vi "Read Properties.vi"(11 "Grid in":refnum<class "Grid.lvclass">) -> (0 "No Neurons":i32, 1 "Neurons Info":T1, 2 "Size(um)":u32[](array[numeric]), 3 "Grid out":refnum<class "Grid.lvclass">, 4 "Created at":timestamp, 5 "Name XML File":string, 6 "Comments":string, 7 "Path":path)   [LabVIEW 2013, in "Grid.lvclass"]
doc: "This VI gets the global information of the grid: No Neurons, Neurons Info, and Size Cube"
uses:
  Grid.lvclass
  Controls/Neuron Info.ctl
  Controls/Type of Neuron.ctl
  Grid.lvclass/Grid.ctl
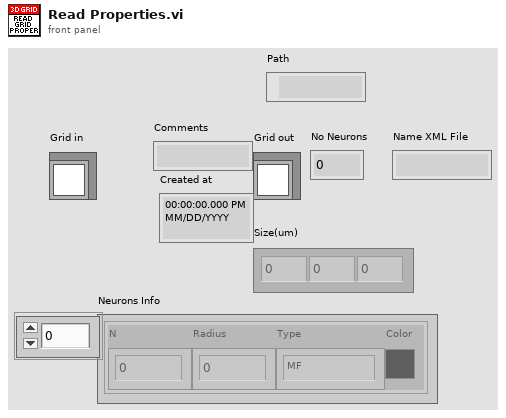
[diagram p1: front panel]
types:
  T1 = typedef "Neuron Info.ctl" = cluster{"N":i32, "Radius":dbl, "Type":T2, "Color":u32}[]
  T2 = typedef "Type of Neuron.ctl" = enum16{"MF", "BA", "GO", "GC", "PC", "LU", "Glia (Dummy)"}
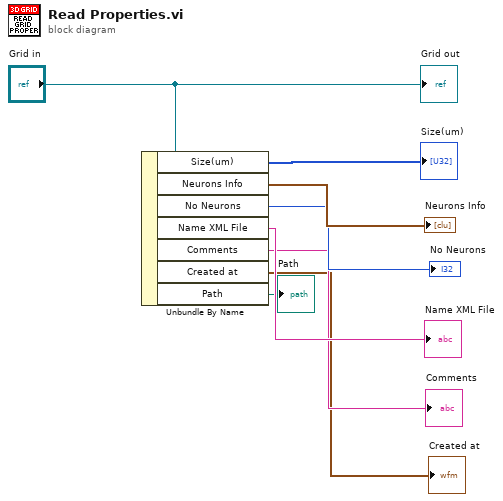
[diagram p0: block diagram]
diagram:
  n1 = Unbundle By Name("Grid in") -> ("Size(um)"=→"Size(um)":u32[], "Neurons Info"=→"Neurons Info":T1, "No Neurons"=→"No Neurons":i32, "Name XML File"=→"Name XML File":string, "Comments"=→"Comments":string, "Created at"=→"Created at":timestamp, "Path"=→"Path":path)
  "Grid out" <- "Grid in"
